vi "HeaterAlarmStatusChanged.vi"(7 "ControlQueue":refnum<queue>, 8 "entrée d'erreur (pas d'erreur)":errorcluster, 9 "HeaterAlarmStatus":bool, 10 "HeaterAlarmStatusChanged":bool, 11 "DAQmxTaskContainer en entrée":refnum<class "DAQmxTaskContainer.lvclass">) -> (0 "sortie d'erreur":errorcluster, 2 "Alarm":bool, 3 "DAQmxTaskContainer en sortie":refnum<class "DAQmxTaskContainer.lvclass">)   [LabVIEW 2015, in "DAQmxTaskContainer.lvclass"]
uses:
  DAQmxTaskContainer.lvclass
  DAQmxTaskContainer_General/DAQmxTaksContainer_General.lvclass/DAQmxTaksContainer_General.ctl
  dependecies/ControlsVIs/Clusters-def/Standard Command.ctl
  dependecies/ControlsVIs/Clusters-def/SERVER-Commands.ctl
  dependecies/ControlsVIs/Clusters-def/ProtypeCommand-DAQmxReply.ctl
  dependecies/ControlsVIs/Clusters-def/Message types.ctl
  DAQmxTask.lvclass
  Control/Control-Server/Control-Server.lvclass
  Message/Message.lvclass
  GeneralFunctionality/GeneralFunctionality.lvclass
  DAQmxTaskContainer_General/DAQmxTaksContainer_General.lvclass
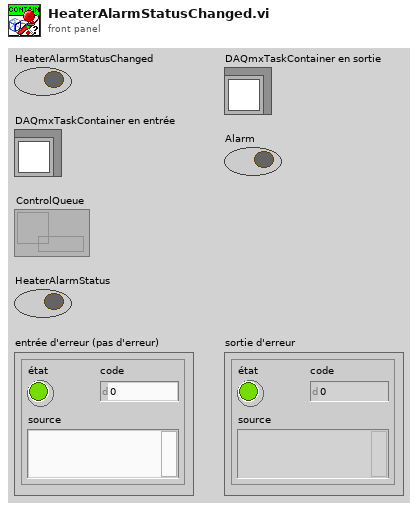
[diagram p1: front panel]
types:
  T1 = typedef "Message types.ctl" = string
  T2 = typedef "ProtypeCommand-DAQmxReply.ctl" = cluster{"On/Off":bool, "error out":errorcluster}
  T3 = typedef "Control-Server.lvclass/SERVER-Commands.ctl" = string
  T4 = typedef "Standard Command.ctl" = cluster{"command":string, "data":variant}
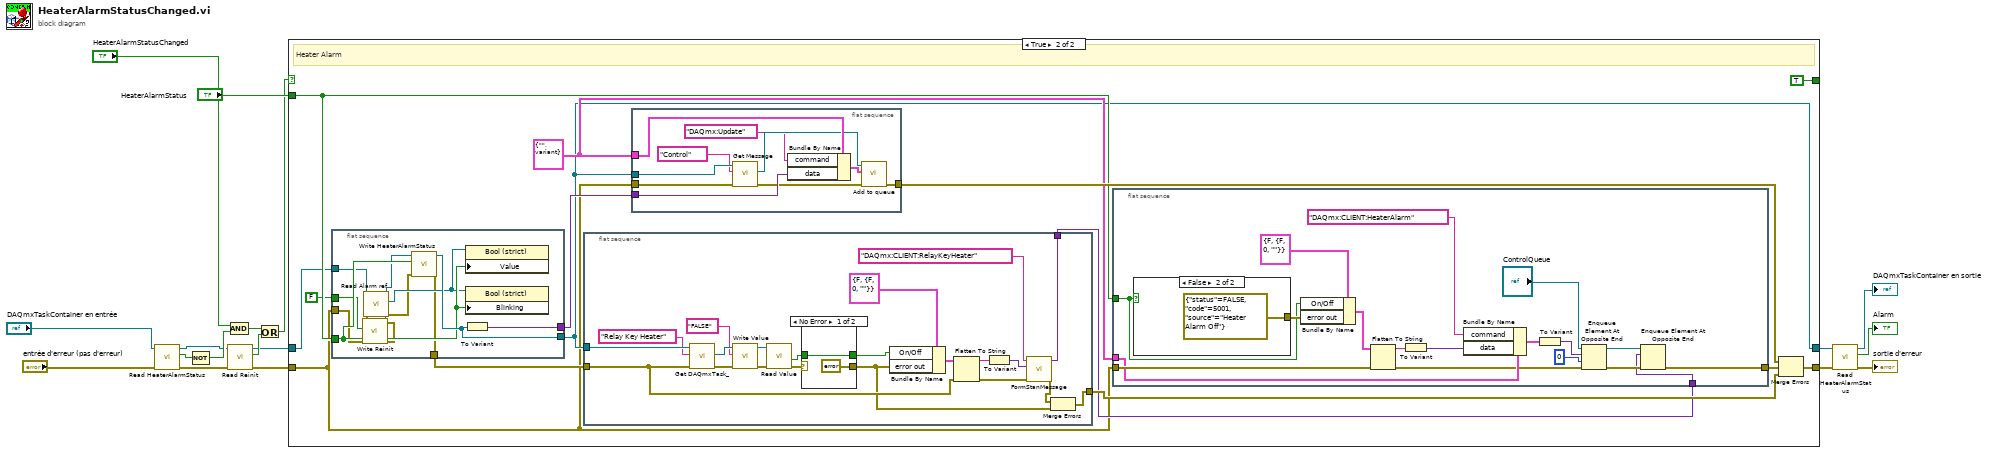
[diagram p0: block diagram]
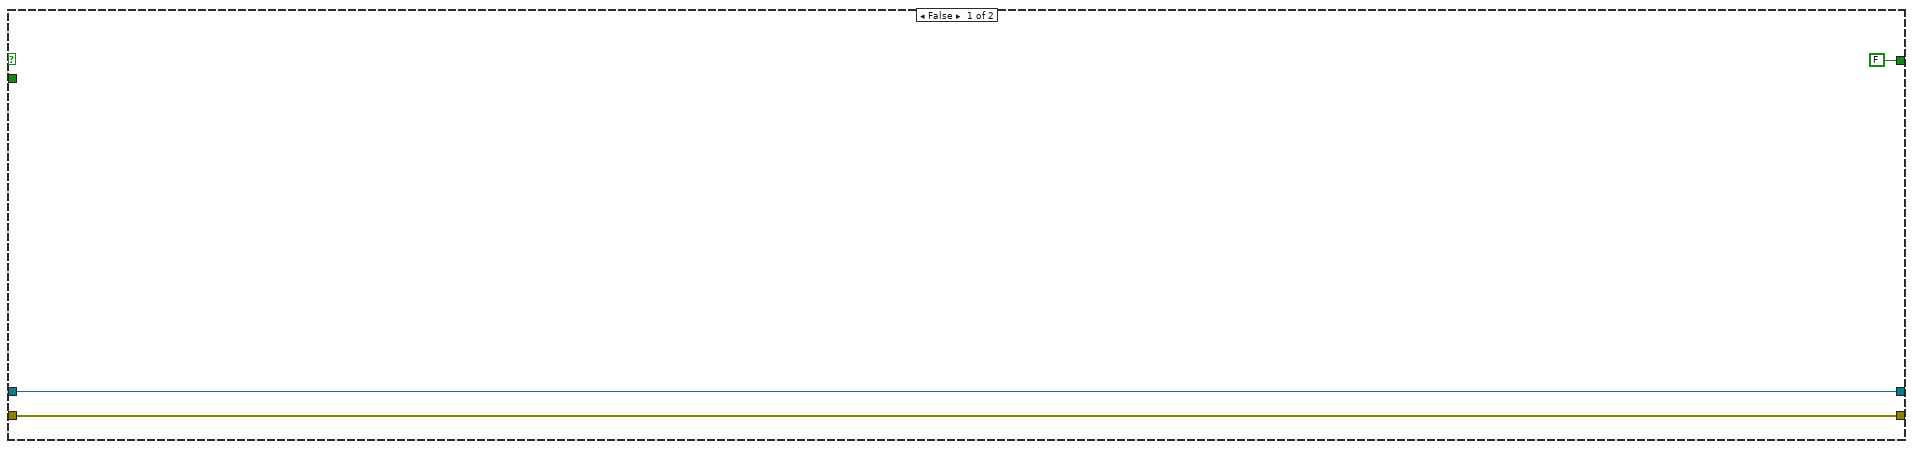
[diagram p2: hidden frame]
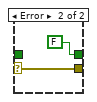
[diagram p3: hidden frame]
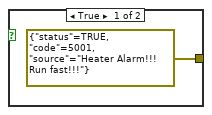
[diagram p4: hidden frame]
diagram:
  n1 = call "Read HeaterAlarmStatus.vi"("error in (no error)"="entrée d'erreur (pas d'erreur)", "DAQmxTaksContainer_General in"="DAQmxTaskContainer en entrée") -> ("error out"=w10:errorcluster, "HeaterAlarmStatus"=w13:bool, "DAQmxTaksContainer_General out"=w7:refnum<class "DAQmxTaskContainer.lvclass">)  [unwired: 7 in]
  n2 = Not(x=w13) -> (.not. x?=w16:bool)
  n3 = And(x="HeaterAlarmStatusChanged", y=w16) -> (x .and. y?=w15:bool)
  n4 = call "Read Reinit.vi"("error in (no error)"=w10, "DAQmxTaksContainer_General in"=w7) -> ("error out"=w9:errorcluster, "Reinit"=w12:bool, "DAQmxTaksContainer_General out"=w6:refnum<class "DAQmxTaskContainer.lvclass">)  [unwired: 7 in]
  n5 = Or(x=w15, y=w12) -> (x .or. y?=w14:bool)
  n6 = case shown="True" w14 {
    tunnel: [w21 w34] -> w5
    tunnel: [FALSE ("Alarm") TRUE ("Alarm")] -> _
    tunnel: w6 -> [w19 w25]
    tunnel: w9 -> [w21 w22]
    tunnel: [w19 w27] -> w2
    tunnel: "HeaterAlarmStatus" -> [_ w29]
    frame False {
    }
    frame True {
      w32 = T4 {"command"="", "data"=variant} ("input cluster")
      # "Heater Alarm"
      n7 = flat-sequence {
        tunnel: [w47] -> w31
        tunnel: w29 -> [w45]
        tunnel: [w46] -> w27
        tunnel: w25 -> [w38]
        tunnel: [w41] -> w24
        tunnel: FALSE ("AlarmOccured") -> [w40]
        tunnel: w22 -> [w36]
        frame #0 {
          n8 = call "Write Reinit.vi"("error in (no error)"=w36, "Reinit"=w40, "DAQmxTaksContainer_General in"=w38) -> ("error out"=w39:errorcluster, "DAQmxTaksContainer_General out"=w37:refnum<class "DAQmxTaskContainer.lvclass">)  [unwired: 7 in]
          n9 = call "Read Alarm ref.vi"("error in (no error)"=w39, "DAQmxTaksContainer_General in"=w37) -> ("error out"=w43:errorcluster, "Alarm"=w44:refnum<vi>, "DAQmxTaksContainer_General out"=w42:refnum<class "DAQmxTaskContainer.lvclass">)  [unwired: 7 in]
          n10 = call "Write HeaterAlarmStatus.vi"("error in (no error)"=w43, "HeaterAlarmStatus"=w45, "DAQmxTaksContainer_General in"=w42) -> ("error out"=w41:errorcluster, "DAQmxTaksContainer_General out"=w46:refnum<class "DAQmxTaskContainer.lvclass">)  [unwired: 7 in]
          n11 = To Variant(anything=w46) -> (Variant=w47:variant)
          n12 = property on="Property Node" class="Bool (strict)"(reference=w44, "Value"=w45) -> ()  [unwired: 1 in, 2 out]
          n13 = property on="Property Node" class="Bool (strict)"(reference=w44, "Blinking"=w45) -> ()  [unwired: 1 in, 2 out]
        }
      }
      n14 = flat-sequence {
        tunnel: w24 -> [w61]
        tunnel: w27 -> [w78]
        tunnel: [w59] -> w28
        tunnel: [w62] -> w26
        frame #0 {
          n15 = call "Get DAQmxTask_.vi"("error in (no error)"=w61, "Task name"="Relay Key Heater", "DAQmxTaksContainer_General in"=w78) -> ("error out"=w76:errorcluster, "DAQmx Task"=w77:refnum<class "DAQmxTask.lvclass">)  [unwired: 6 in, 1 out]
          n16 = call-dynamic "Write Value.vi"("error in (no error)"=w76, "Data"="FALSE", "DAQmxTask en entrée"=w77) -> ("error out"=w73:errorcluster, "DAQmxTask en sortie"=w72:refnum<class "DAQmxTask.lvclass">)  [unwired: 7 in]
          n17 = call-dynamic "Read Value.vi"("error in (no error)"=w73, "DAQmxTask en entrée"=w72) -> ("error out"=w65:errorcluster, "Data"=w64:bool)  [unwired: 6 in, 2 out]
          n18 = case shown="No Error" w65 {
            selector: w65 -> [_ w82]
            tunnel: [errorcluster {"status"=FALSE, "code"=5001, "source"="Relay key heater worked"} ("error constant") w82] -> w58
            tunnel: w64 -> [w79 _]
            tunnel: [w79 FALSE] -> w63
            frame No Error {
            }
            frame Error {
            }
          }
          n19 = Bundle By Name(cluster=T2 {"On/Off"=FALSE, "error out"={"status"=FALSE, "code"=0, "source"=""}} ("output cluster"), "On/Off"=w63, "error out"=w58) -> (w68:T2)
          n20 = Flatten To String(anything=w68, error in (no error)=w61) -> (data string=w67:string, error out=w71:errorcluster)  [unwired: 2 in, 1 out]
          n21 = To Variant(anything=w67) -> (Variant=w70:variant)
          n22 = call "FormStanMessage.vi"("error in"=w71, "data"=w70, "Command"=T3 "DAQmx:CLIENT:RelayKeyHeater" ("command")) -> ("error out"=w60:errorcluster, "message"=w62:variant)  [unwired: 7 in]
          n23 = Merge Errors(w60, w58) -> (w59:errorcluster)
        }
      }
      n24 = flat-sequence {
        tunnel: w22 -> [w57]
        tunnel: [w56] -> w33
        tunnel: w32 -> [w55]
        tunnel: w31 -> [w54]
        tunnel: w27 -> [w53]
        frame #0 {
          n25 = call "Get Message.vi"("error in (no error)"=w57, "Message type"=T1 "Control", "GeneralFunctionality en entrée"=w53) -> ("error out"=w51:errorcluster, "Message.lvclass"=w52:refnum<class "Message.lvclass">)  [unwired: 6 in, 1 out]
          n26 = Bundle By Name(cluster=w55, "command"="DAQmx:Update", "data"=w54) -> (w49:T4)
          n27 = call "Add to queue.vi"("error in (no error)"=w51, "Data"=w49, "Message in"=w52) -> ("error out"=w56:errorcluster)  [unwired: 7 in, 1 out]
        }
      }
      n28 = flat-sequence {
        tunnel: w22 -> [w94]
        tunnel: w32 -> [w93]
        tunnel: [w84] -> w30
        tunnel: w29 -> [w89]
        tunnel: w26 -> [w83]
        frame #0 {
          n29 = case shown="False" w89 {
            tunnel: [errorcluster {"status"=TRUE, "code"=5001, "source"="Heater Alarm!!! Run fast!!!"} ("error out") errorcluster {"status"=FALSE, "code"=5001, "source"="Heater Alarm Off"} ("error out")] -> w96
            frame True {
            }
            frame False {
            }
          }
          n30 = Bundle By Name(cluster=T2 {"On/Off"=FALSE, "error out"={"status"=FALSE, "code"=0, "source"=""}} ("output cluster"), "On/Off"=w89, "error out"=w96) -> (w97:T2)
          n31 = Flatten To String(anything=w97, error in (no error)=w94) -> (data string=w100:string, error out=w87:errorcluster)  [unwired: 2 in, 1 out]
          n32 = To Variant(anything=w100) -> (Variant=w99:variant)
          n33 = Bundle By Name(cluster=w93, "command"=T3 "DAQmx:CLIENT:HeaterAlarm" ("Command"), "data"=w99) -> (w98:T4)
          n34 = To Variant(anything=w98) -> (Variant=w91:variant)
          n35 = Enqueue Element At Opposite End(queue="ControlQueue", element=w91, timeout in ms (-1)=0 ("timeout en ms (-1)"), error in (no error)=w87) -> (queue out=w85:refnum<queue>, error out=w86:errorcluster)  [unwired: 1 out]
          n36 = Enqueue Element At Opposite End(queue=w85, element=w83, error in (no error)=w86) -> (error out=w84:errorcluster)  [unwired: 1 in, 2 out]
        }
      }
      n37 = Merge Errors(w33, w30, w28) -> (w34:errorcluster)
    }
  }
  n38 = call "Read HeaterAlarmStatus.vi"("error in (no error)"=w5, "DAQmxTaksContainer_General in"=w2) -> ("error out"=→"sortie d'erreur":errorcluster, "HeaterAlarmStatus"=→"Alarm":bool, "DAQmxTaksContainer_General out"=→"DAQmxTaskContainer en sortie":refnum<class "DAQmxTaskContainer.lvclass">)  [unwired: 7 in]
